vi "calcUkRefX0.vi"(8 "error in (no error)":errorcluster, 10 "Qx Array":dbl[][](array[numeric]), 11 "OptCtrl in":refnum<class "OptCtrl.lvclass">) -> (0 "error out":errorcluster, 2 "uk Array":dbl[](array[numeric]), 3 "OptCtrl out":refnum<class "OptCtrl.lvclass">)   [LabVIEW 2016, in "OptCtrl.lvclass"]
doc: "Calculate uk by referencing to \"x0\". The offset will only trace the previous one."
uses:
  OptCtrl.lvclass
  OptCtrl.lvclass/OptCtrl.ctl
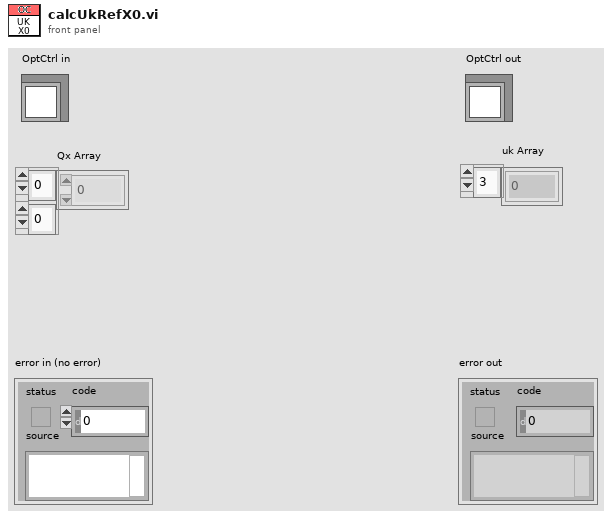
[diagram p1: front panel]
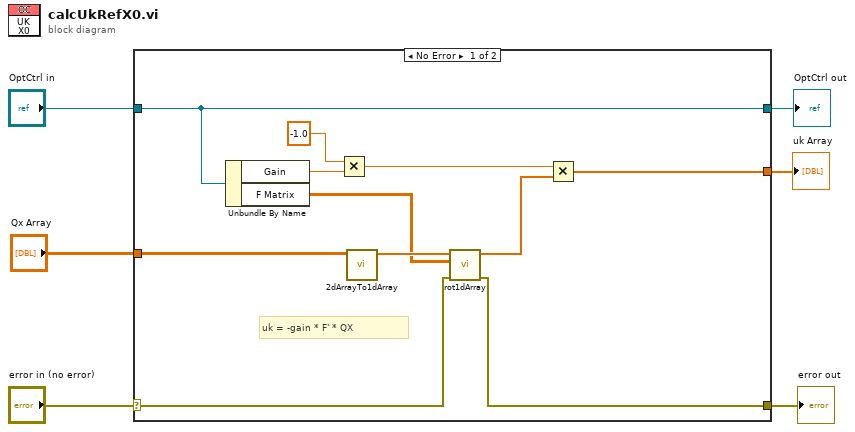
[diagram p0: block diagram]
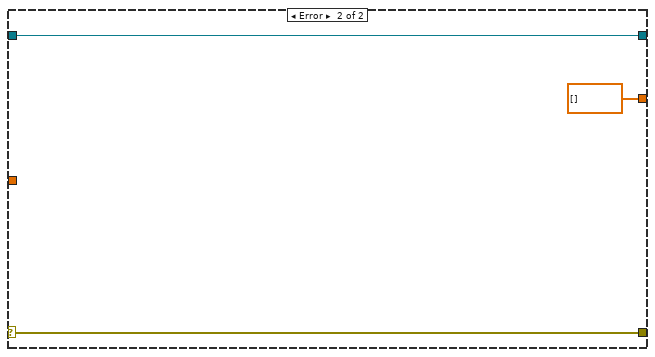
[diagram p2: hidden frame]
diagram:
  n1 = case shown="No Error" "error in (no error)" {
    selector: "error in (no error)" -> [w11 w20]
    tunnel: [w10 w20] -> w5
    tunnel: [w17 w19] -> w3
    tunnel: "OptCtrl in" -> [w17 w19]
    tunnel: "Qx Array" -> [w13 _]
    tunnel: [w7 dbl[] [] ("1D Array")] -> w1
    frame No Error {
      # "uk = -gain * F' * QX"
      n2 = Unbundle By Name(w17) -> ("Gain"=w15:dbl, "F Matrix"=w9:dbl[][])
      n3 = Multiply(x=-1.0, y=w15) -> (x*y=w14:dbl)
      n4 = call "2dArrayTo1dArray.vi"("2D Array"=w13) -> ("1D Array"=w12:dbl[])  [unwired: 10 in]
      n5 = call "rot1dArray.vi"("error in (no error)"=w11, "Rot Mat"=w9, "1D Array"=w12) -> ("error out"=w10:errorcluster, "Rotated 1D Array"=w8:dbl[])  [unwired: 7 in]
      n6 = Multiply(x=w14, y=w8) -> (x*y=w7:dbl[])
    }
    frame Error {
    }
  }
  "error out" <- w5
  "OptCtrl out" <- w3
  "uk Array" <- w1
